vi "MSEncoder SubVI Press2Continue.vi"(7 "error in (no error)":errorcluster, 9 "Boolean in":refnum<vi>) -> (0 "error out":errorcluster)   [LabVIEW 2018]
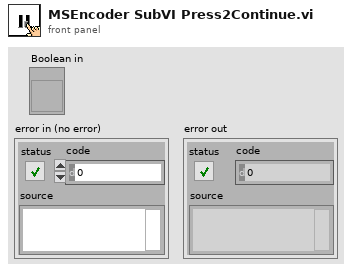
[diagram p1: front panel]
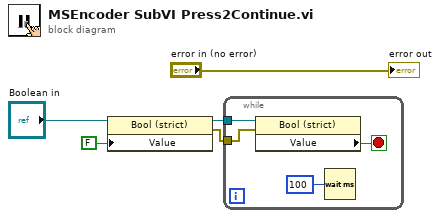
[diagram p0: block diagram]
diagram:
  n1 = property class="Bool (strict)"(reference="Boolean in", "Value"=FALSE) -> (reference out=w4:refnum<vi>, error out=w2:errorcluster)  [unwired: 1 in]
  n2 = while {
    tunnel: w4 -> [w9]
    tunnel: w2 -> [w6]
    stop <- w8 stop-if-true
    n3 = property class="Bool (strict)"(reference=w9, error in=w6) -> ("Value"=w8:bool)  [unwired: 2 out]
    n4 = Wait (ms)(milliseconds to wait=u32 100) -> ()  [unwired: 1 out]
  }
  "error out" <- "error in (no error)"
